vi "TelemetryServer_MultiplexerStart.vi"(2 "Multiplexer Group":string, 3 "Telemetry":string[](array[string]), 9 "Error in (no error)":errorcluster caption="error in (no error)") -> (0 "Multiplexer":T1, 6 "Error out":errorcluster caption="error out")   [LabVIEW 2009]
uses:
  TelemetryServer_Global.vi
panel:
  in  "élément":waveform(dbl)={"t0"=timestamp(0 s since 1904-01-01), "dt"=0.0, "Y"=[]}
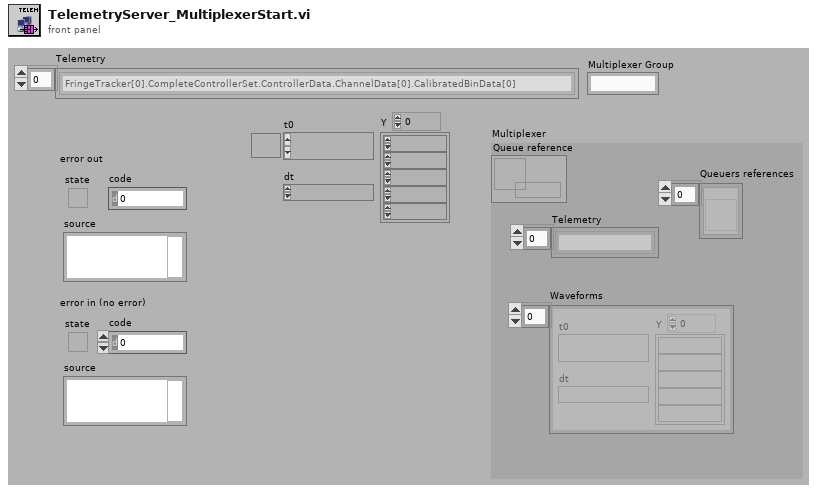
[diagram p1: front panel]
types:
  T1 = cluster{"Queue reference":refnum<queue>, "Telemetry":string[], "Queuers references":refnum<vi>[], "Waveforms":waveform(dbl)[]}
  T2 = cluster{"queue out":refnum<queue>, string[], refnum<vi>[], waveform(dbl)[]}
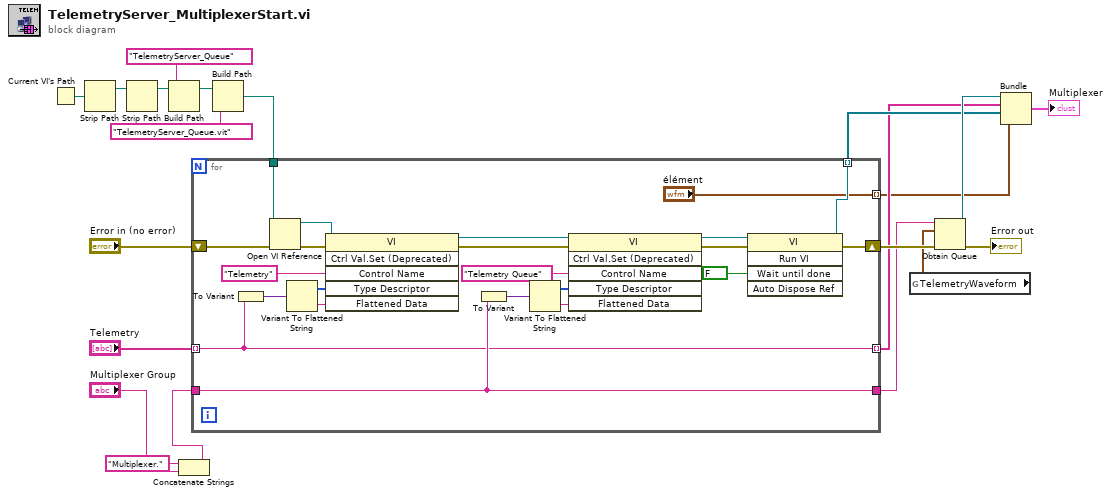
[diagram p0: block diagram]
diagram:
  n1 = Current VI's Path() -> (path=w20:path)
  n2 = Strip Path(path=w20) -> (stripped path=w13:path)  [unwired: 1 out]
  n3 = Strip Path(path=w13) -> (stripped path=w11:path)  [unwired: 1 out]
  n4 = Build Path(base path=w11, name or relative path="TelemetryServer_Queue" ("nom ou chemin relatif")) -> (appended path=w9:path)
  n5 = Concatenate Strings("Multiplexer." ("chaîne"), "Multiplexer Group") -> (w2:string)
  n6 = Build Path(base path=w9, name or relative path="TelemetryServer_Queue.vit" ("nom ou chemin relatif")) -> (appended path=w19:path)
  n7 = for {
    tunnel: "Telemetry" -> [w24] mode=indexing
    tunnel: w2 -> [w25]
    tunnel: w19 -> [w26]
    shift-right: [w27] -> w17
    shift-left: "Error in (no error)" -> [w28]
    tunnel: [w25] -> w15
    tunnel: [w24] -> w5 mode=indexing
    tunnel: [w23] -> w6 mode=indexing
    tunnel: ["élément"] -> w1 mode=indexing
    n8 = To Variant(anything=w24) -> (Variant=w39:variant)
    n9 = Open VI Reference(vi path=w26, error in (no error)=w28) -> (vi reference=w42:refnum<vi>, error out=w43:errorcluster)  [unwired: 4 out]
    n10 = Variant To Flattened String(Variant=w39) -> (data string=w40:string, 1:w41:i16[])
    n11 = invoke class="VI" method="Ctrl Val.Set (Deprecated)"(reference=w42, error in=w43, "Control Name"="Telemetry" ("Nom de la commande"), "Type Descriptor"=w41, "Flattened Data"=w40) -> (reference out=w32:refnum<vi>, error out=w33:errorcluster)  [unwired: 1 in, 4 out]
    n12 = To Variant(anything=w25) -> (Variant=w36:variant)
    n13 = Variant To Flattened String(Variant=w36) -> (data string=w35:string, 1:w34:i16[])
    n14 = invoke class="VI" method="Ctrl Val.Set (Deprecated)"(reference=w32, error in=w33, "Control Name"="Telemetry Queue" ("Nom de la commande"), "Type Descriptor"=w34, "Flattened Data"=w35) -> (reference out=w30:refnum<vi>, error out=w31:errorcluster)  [unwired: 1 in, 4 out]
    n15 = invoke class="VI" method="Run VI"(reference=w30, error in=w31, "Wait until done"=FALSE ("Attente synchrone")) -> (reference out=w23:refnum<vi>, error out=w27:errorcluster)  [unwired: 2 in, 3 out]
  }
  n16 = global read "TelemetryServer_Global.vi" "TelemetryWaveform"() -> (w14:waveform(dbl))
  n17 = Obtain Queue(name (unnamed)=w15, element data type=w14, error in (no error)=w17) -> (queue out=w8:refnum<queue>, error out=→"Error out":errorcluster)  [unwired: 2 in, 1 out]
  n18 = Bundle("queue out"=w8, w5, w6, w1) -> (→"Multiplexer":T2)  [unwired: 1 out]
